vi "UHR-Fleezers Control (host) -Leonardo 04-2018 V3_greenctrl.vi"(0 "Tab Green FB":T5(tab)=enum."Trap Control (RF)") -> ()   [LabVIEW 2013] (continued)
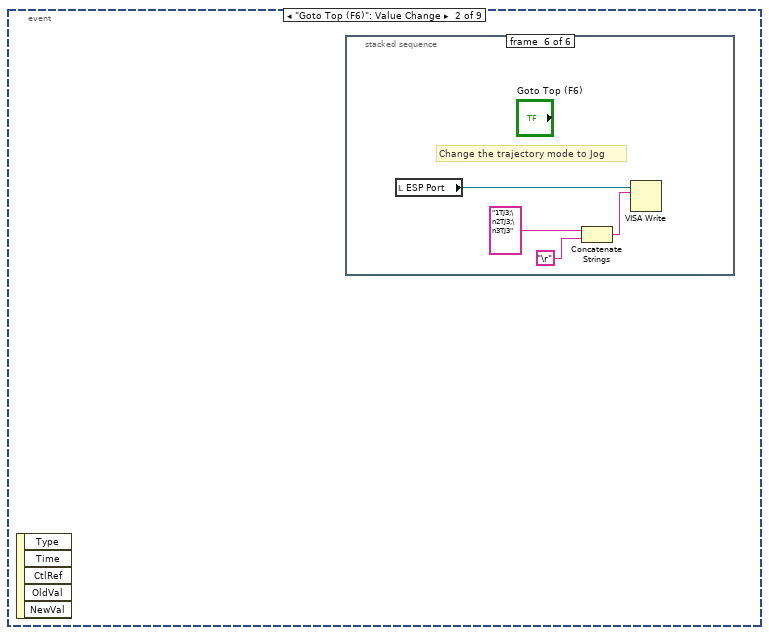
[diagram p4: hidden frame]
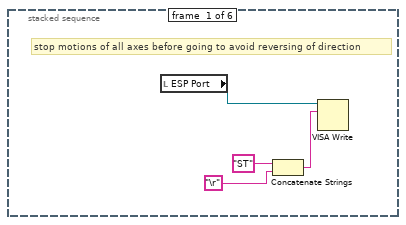
[diagram p5: hidden frame]
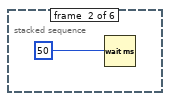
[diagram p6: hidden frame]
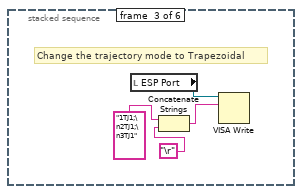
[diagram p7: hidden frame]
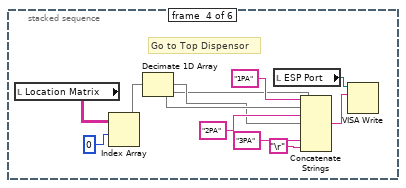
[diagram p8: hidden frame]
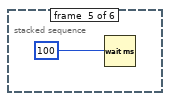
[diagram p9: hidden frame]
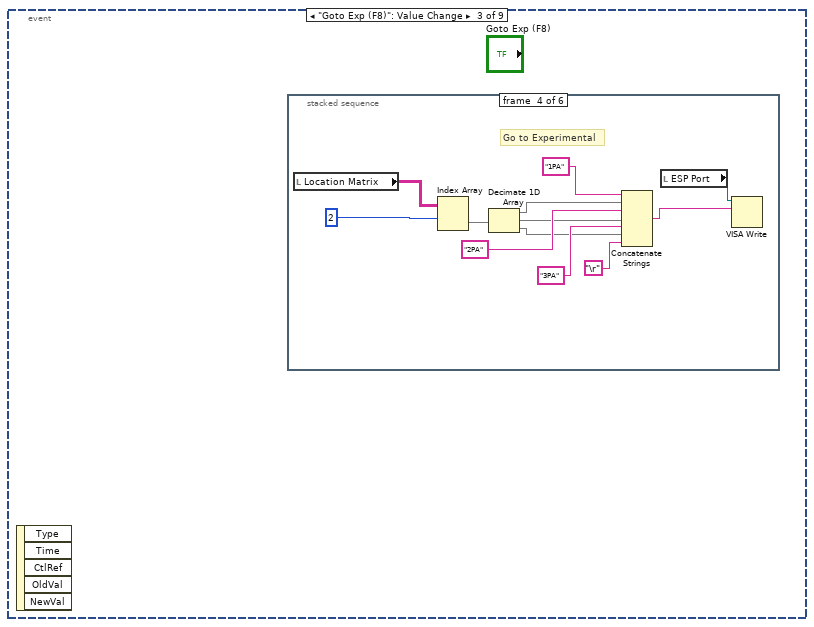
[diagram p10: hidden frame]
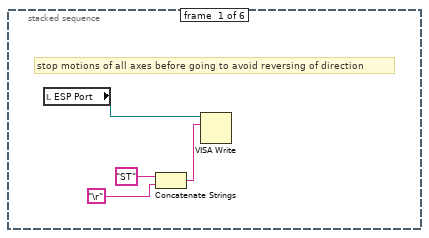
[diagram p11: hidden frame]
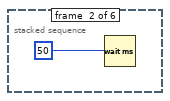
[diagram p12: hidden frame]
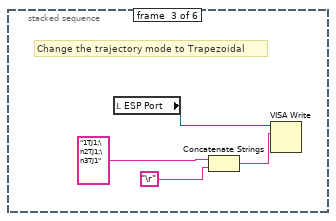
[diagram p13: hidden frame]
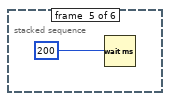
[diagram p14: hidden frame]
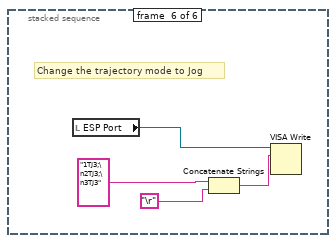
[diagram p15: hidden frame]
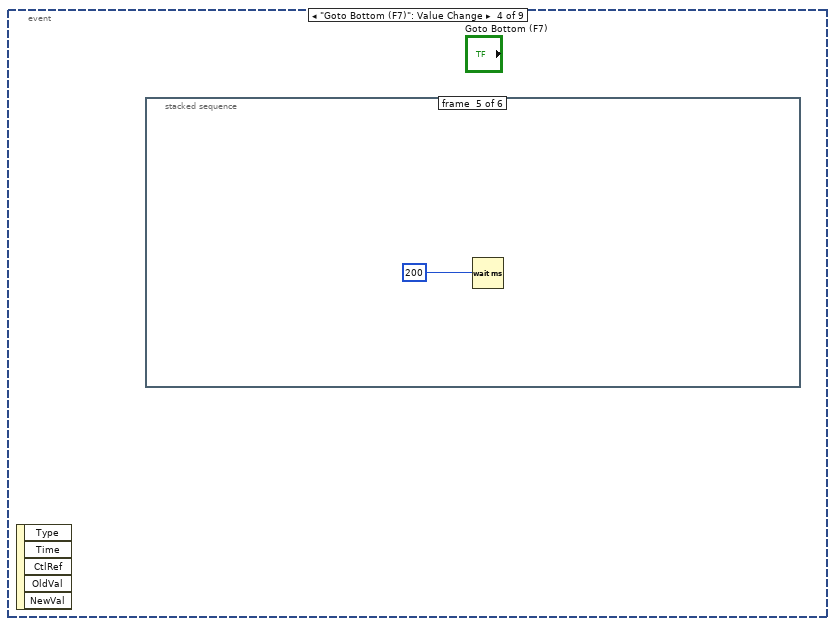
[diagram p16: hidden frame]
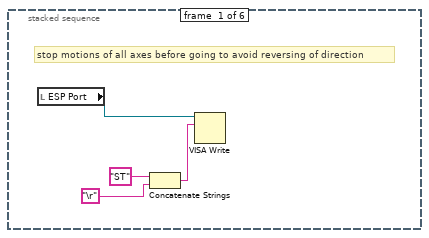
[diagram p17: hidden frame]
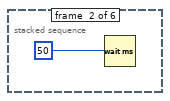
[diagram p18: hidden frame]
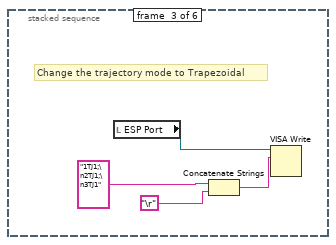
[diagram p19: hidden frame]
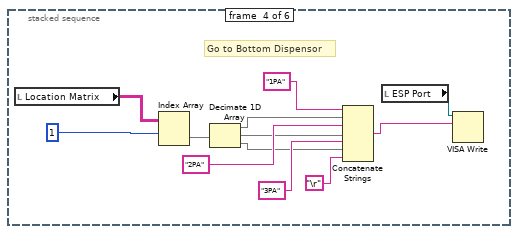
[diagram p20: hidden frame]
                  tunnel: w3888 -> [w3958 w3969]
                  tunnel: [w3958 w3961] -> w3887
                  tunnel: "Save ave N" -> [_ w3962]
                  frame False {
                  }
                  frame True {
                    w3959 = 2 ("dimension size")
                    n2326 = Array Size(array=w3969) -> (size(s)=w3963:i32)
                    n2327 = Divide(x=w3963, y=w3959) -> (x/y=w3967:dbl)
                    n2328 = Reshape Array(w3969, w3967, w3959) -> (w3968:u64[][])
                    n2329 = Transpose 2D Array(2D array=w3968) -> (transposed array=w3966:u64[][])
                    n2330 = for {
                      tunnel: w3966 -> [w3971] mode=indexing
                      tunnel: [w3970] -> w3960 mode=indexing
                      tunnel: w3962 -> [w3972]
                      workers-P: _ -> [_]
                      n2331 = call "downsample 1D array - U64.vi"("Ave N"=w3972, "Array In"=w3971) -> ("Array Out"=w3970:u64[])  [unwired: 1 in]
                    }
                    n2332 = Transpose 2D Array(2D array=w3960) -> (transposed array=w3965:u64[][])
                    n2333 = Divide(x=w3963, y=w3962) -> (x/y=w3964:dbl)
                    n2334 = Reshape Array(w3965, w3964) -> (w3961:u64[])
                  }
                }
                n2335 = case shown="True" w3889 {
                  tunnel: w3949 -> [w3981 w3993]
                  tunnel: [w3981 w3985] -> w3945
                  tunnel: "Save ave N" -> [_ w3986]
                  tunnel: w3940 -> [_ w3984]
                  frame False {
                    # "don't downsample data for trap calibration"
                  }
                  frame True {
                    n2336 = Array Size(array=w3993) -> (size(s)=w3987:i32)
                    n2337 = Array Size(array=w3984) -> (size(s)=w3983:i32)
                    n2338 = Divide(x=w3987, y=w3983) -> (x/y=w3991:dbl)
                    n2339 = Reshape Array(w3993, w3991, w3983) -> (w3992:i16[][])
                    n2340 = Transpose 2D Array(2D array=w3992) -> (transposed array=w3990:i16[][])
                    n2341 = for {
                      tunnel: w3990 -> [w3996] mode=indexing
                      tunnel: [w3995] -> w3982 mode=indexing
                      tunnel: w3986 -> [w3994]
                      workers-P: _ -> [_]
                      n2342 = call "downsample 1D array - I16.vi"("Ave N"=w3994, "Array In"=w3996) -> ("Array Out"=w3995:i16[])  [unwired: 1 out]
                    }
                    n2343 = Transpose 2D Array(2D array=w3982) -> (transposed array=w3989:i16[][])
                    n2344 = Divide(x=w3987, y=w3986) -> (x/y=w3988:dbl)
                    n2345 = Reshape Array(w3989, w3988) -> (w3985:i16[])
                  }
                }
                n2346 = Index Array(array=w3911, index=1) -> (element=w3914:waveform(dbl))
                n2347 = Index Array(array=w3911, index=0) -> (element=w3916:waveform(dbl))
                n2348 = Unbundle By Name(w3914) -> ("Y"=w3918:dbl[])
                n2349 = Unbundle By Name(w3916) -> ("Y"=w3926:dbl[])
                n2350 = case "Write trap pos. data" shown="True" w3892 {
                  tunnel: w3891 -> [_ w3974]
                  tunnel: w3887 -> [_ w3973]
                  frame False {
                  }
                  frame True {
                    n2351 = Write to Binary File(file (use dialog)=w3974, data=w3973, 5:FALSE ("prepend array or string size? (T)"), 9:T30."big-endian, network order" ("byte order (0:big-endian, network order)")) -> ()  [unwired: 1 in, 4 out]
                  }
                }
                n2352 = Write to Binary File(file (use dialog)=w3952, data=w3945, 5:FALSE ("prepend array or string size? (T)"), 9:T30."big-endian, network order" ("byte order (0:big-endian, network order)")) -> ()  [unwired: 1 in, 4 out]
                n2353 = feedback #26(w3918) -> (w3920:dbl[])
                n2354 = Build Array (concatenate)(w3920, w3918) -> (w3919:dbl[])
                n2355 = Select(t=w3918, s=w3894, f=w3919) -> (s? t:f=w3904:dbl[])
                n2356 = feedback-in #26(w3904) -> ()
                n2357 = feedback #27(w3926) -> (w3939:dbl[])
                n2358 = Build Array (concatenate)(w3939, w3926) -> (w3938:dbl[])
                n2359 = Select(t=w3926, s=w3894, f=w3938) -> (s? t:f=w3913:dbl[])
                n2360 = feedback-in #27(w3913) -> ()
                n2361 = Divide(x=w3953, y=w3954) -> (x/y=w3956:dbl)
                n2362 = Multiply(x=w3956, y=100.0) -> (x*y=w3955:dbl)
                n2363 = Build Array(w3913, w3904) -> (→"Saved APD":dbl[][])
                n2364 = Array Size(array=w3913) -> (size(s)=w3931:i32)
                n2365 = Unbundle By Name(w3933) -> ("Y"=w3937:dbl[])
                n2366 = Subtract(x=w3931, y="N pts to average") -> (x-y=w3907:i32)
                n2367 = Multiply(x="N pts to average", y=u16 2) -> (x*y=w3908:u16)
                n2368 = Subtract(x=w3931, y=w3908) -> (x-y=w3906:i32)
                n2369 = feedback #28(w3937) -> (w3936:dbl[])
                n2370 = Build Array (concatenate)(w3936, w3937) -> (w3935:dbl[])
                n2371 = Select(t=w3937, s=w3894, f=w3935) -> (s? t:f=w3934:dbl[])
                "Trap Delta Graph" <- w3934
                n2372 = feedback-in #28(w3934) -> ()
                n2373 = Array Subset(array=w3913, index=w3907, length="N pts to average") -> (w3930:dbl[])
                n2374 = Array Subset(array=w3913, index=w3906, length="N pts to average") -> (w3929:dbl[])
                n2375 = Array Subset(array=w3904, index=w3907, length="N pts to average") -> (w3910:dbl[])
                n2376 = Array Subset(array=w3904, index=w3906, length="N pts to average") -> (w3909:dbl[])
                n2377 = call-poly <vilib>:"Mean.vi"("X"=w3930) -> ("mean"=w3928:dbl)  [unwired: 1 out]
                n2378 = call-poly <vilib>:"Mean.vi"("X"=w3910) -> ("mean"=w3903:dbl)  [unwired: 1 out]
                n2379 = call-poly <vilib>:"Mean.vi"("X"=w3929) -> ("mean"=w3927:dbl)  [unwired: 1 out]
                n2380 = call-poly <vilib>:"Mean.vi"("X"=w3909) -> ("mean"=w3902:dbl)  [unwired: 1 out]
                n2381 = Subtract(x=w3903, y=w3902) -> (x-y=w3893:dbl)
                "Delta Fl. 2" <- w3893
                n2382 = Subtract(x=w3928, y=w3927) -> (x-y=w3925:dbl)
                "Delta Fl. 1" <- w3925
                n2383 = Initialize Array(w3925, 1 ("dimension size")) -> (w3922:dbl[])
                n2384 = Initialize Array(w3893, 1 ("dimension size")) -> (w3899:dbl[])
                n2385 = feedback #29(w3922) -> (w3923:dbl[])
                n2386 = Build Array (concatenate)(w3923, w3922) -> (w3921:dbl[])
                n2387 = feedback #30(w3899) -> (w3900:dbl[])
                n2388 = Build Array (concatenate)(w3900, w3899) -> (w3898:dbl[])
                n2389 = Select(t=w3922, s=w3894, f=w3921) -> (s? t:f=w3897:dbl[])
                n2390 = feedback-in #29(w3897) -> ()
                n2391 = Select(t=w3899, s=w3894, f=w3898) -> (s? t:f=w3896:dbl[])
                n2392 = feedback-in #30(w3896) -> ()
                n2393 = Build Array(w3897, w3896) -> (→"Save APD Deriv":dbl[][])
              }
            }
            "Progress" <- w3870
            "Progress 2" <- w3870
          }
        }
      }
    }
    n2394 = Divide(x=w2251, y=w2252) -> (x/y=w2242:ext)
    "Trap 2 amplitude" <- w2242
    n2395 = Bundle By Name(cluster=w2505, "Green FB Ch 0"=w2504, "Green FB Ch 1"=w2503) -> (w2489:T49)
    "Green FB Signals (V)" <- w2489
    n2396 = case shown="True" w2244 {
      tunnel: w2243 -> [_ w2594]
      tunnel: w2242 -> [_ w2593]
      frame False {
      }
      frame True {
        w2595 = 50.0
        n2397 = Greater?(x=w2593, y=w2595) -> (0:w2591:bool)
        n2398 = Greater?(x=w2594, y=w2595) -> (0:w2592:bool)
        n2399 = Or(x=w2592, y=w2591) -> (x .or. y?=w2590:bool)
        n2400 = case shown="True" w2590 {
          frame False {
          }
          frame True {
            n2401 = property on="All FB On/Off" class="Bool (strict)"("Val(Sgnl)"=FALSE) -> ()  [unwired: 2 in, 2 out]
            "Feedback overload" <- TRUE
          }
        }
      }
    }
    n2402 = Unbundle By Name(w2489) -> ("Green FB Ch 2"=→"Green FB Plot":dbl)
    n2403 = local read "wait to reset values"() -> (w2573:bool)
    n2404 = Not(x=w2570) -> (.not. x?=w2574:bool)
    n2405 = And(x=w2574, y=w2573) -> (x .and. y?=w2575:bool)
    n2406 = case "Part of MCL raster scanning: returns to initial positions after scan done" shown="True" w2575 {
      tunnel: w2578 -> [w3419 w3426]
      tunnel: [w3419 w3425] -> w2577
      tunnel: w2572 -> [w3418 w3424]
      tunnel: [w3418 w3423] -> w2571
      frame False {
      }
      frame True {
        w3434 = 10.0 ("y")
        w3433 = 32767.0 ("y")
        # "to return scan values\nafter a synchronous \nAOM scan"
        n2407 = local read "AO2"() -> (w3427:dbl)
        n2408 = local read "AO1"() -> (w3428:dbl)
        n2409 = local write "wait to reset values"(FALSE ("wait to reset values")) -> ()
        n2410 = Multiply(x=w3428, y=w3433) -> (x*y=w3430:dbl)
        n2411 = Multiply(x=w3427, y=w3433) -> (x*y=w3432:dbl)
        n2412 = Divide(x=w3430, y=w3434) -> (x/y=w3429:dbl)
        n2413 = Divide(x=w3432, y=w3434) -> (x/y=w3431:dbl)
        n2414 = To Word Integer(number=w3429) -> (16bit integer=w3435:i16)
        n2415 = To Word Integer(number=w3431) -> (16bit integer=w3436:i16)
        n2416 = local read "Total Counts (ticks)"() -> (w3420:u32)
        n2417 = xnode "Read/Write Control"("FPGA VI Reference In"=w3426, "error in"=w3424, "AO1 (Y)"=w3435, "AO2 (X)"=w3436, "MCL count"=w3420) -> ("FPGA VI Reference Out"=w3425:T20, "error out"=w3423:errorcluster)
        n2418 = local read "Scan Range (V)\n(of steps)"() -> (w3421:dbl)
        n2419 = property on="Scan Range (V)\n(of steps)" class="DigNum (strict)"("Val(Sgnl)"=w3421) -> ()  [unwired: 2 in, 2 out]
      }
    }
    n2420 = node-c288() -> ()  [unwired: 2 out]
  }
  n2421 = node-c288(3 ("Processor")) -> (w108:T25)  [unwired: 3 out]
  n2422 = timed-loop "Oscillate AOD (debugging)" {
    tunnel: w61 -> [w3998]
    tunnel: [w3997] -> w72
    timing: w108 -> [_]
    timing-out: [_] -> w107
    stop <- w3997 stop-if-true
    n2423 = node-c288() -> ()  [unwired: 2 out]
    n2424 = event shown="[0] \"Oscillate Set 2\", \"Fish for Tether\": Value Change" {
      selector: _ -> [_ _ _]
      dyn-events: _ -> [_ _ _]
      timeout: _ -> [_ _ _]
      tunnel: w3998 -> [w4005 _ _]
      tunnel: [FALSE ("Stop All") _ w4273] -> w3997
      event "Oscillate Set 2", "Fish for Tether": Value Change {
        n2425 = event-data() -> ()  [unwired: 6 out]
        n2426 = local read "Oscillate Set 2"() -> (w4004:bool)
        n2427 = Or(x=w4004, y="Fish for Tether") -> (x .or. y?=w4002:bool)
        n2428 = case shown="True" w4002 {
          tunnel: w4005 -> [_ w4008]
          tunnel: "Fish for Tether" -> [_ w4007]
          frame False {
          }
          frame True {
            n2429 = case shown="True" w4007 {
              frame False {
              }
              frame True {
                n2430 = local write "Scan axis 2"(TRUE) -> ()
                n2431 = local write "Tether"(FALSE ("Tether")) -> ()
              }
            }
            n2432 = node-c288("Period") -> (w4010:T25)  [unwired: 3 out]
            n2433 = timed-loop "Oscillate AOD" {
              timing: w4010 -> [_]
              timing-out: [_] -> w4009
              tunnel: w4008 -> [w4020]
              tunnel: w4007 -> [w4019]
              i -> [w4022]
              stop <- w4018 stop-if-true
              n2434 = node-c288() -> (w4021:i64)  [unwired: 1 out]
              n2435 = flat-sequence {
                tunnel: w4022 -> [w4048]
                tunnel: w4021 -> [w4047]
                tunnel: w4020 -> [w4031]
                tunnel: w4019 -> [w4033]
                tunnel: [w4033] -> w4017
                tunnel: [w4032] -> w4016
                tunnel: [w4030] -> w4015
                tunnel: [w4027] -> w4013
                tunnel: w4017 -> [w4084]
                tunnel: w4016 -> [w4082]
                tunnel: w4015 -> [w4081]
                tunnel: [w4080] -> w4014
                tunnel: w4013 -> [w4079]
                tunnel: [w4148] -> w4018
                tunnel: w4014 -> [w4146]
                frame #0 {
                  n2436 = Divide(x=w4047, y=i64 1000) -> (x/y=w4042:dbl)
                  n2437 = Multiply(x=w4042, y=w4048) -> (x*y=w4044:dbl)
                  n2438 = Multiply(x="Osc. freq. (Hz)", y=6.283185307179586) -> (x*y=w4045:dbl)
                  n2439 = Multiply(x=w4045, y=w4044) -> (x*y=w4029:dbl)
                  n2440 = local read "BD 1 Frequency 2 (MHz)"() -> (w4026:dbl)
                  n2441 = local read "BD 1 Frequency 1 (MHz)"() -> (w4023:dbl)
                  n2442 = case shown="True" w4033 {
                    tunnel: w4029 -> [w4054 w4061]
                    tunnel: w4026 -> [_ w4071]
                    tunnel: [w4051 w4055] -> w4034
                    tunnel: [FALSE w4064] -> w4030
                    tunnel: [0.0 w4057] -> w4027
                    tunnel: w4023 -> [_ w4056]
                    frame False {
                      n2443 = Sine(x=w4054) -> (sin(x)=w4052:dbl)
                      n2444 = Multiply(x=w4052, y="Osc. amp. (MHz)") -> (x*y=w4051:dbl)
                    }
                    frame True {
                      n2445 = Cosine(x=w4061) -> (cos(x)=w4074:dbl)
                      n2446 = Subtract(x=w4071, y=w4056) -> (x-y=w4070:dbl)
                      n2447 = Decrement(x=w4074) -> (x-1=w4073:dbl)
                      n2448 = Subtract(x=w4070, y="Closest Delta (MHz)") -> (x-y=w4067:dbl)
                      n2449 = Divide(x=w4073, y=2.0) -> (x/y=w4068:dbl)
                      n2450 = Multiply(x=w4068, y=w4067) -> (x*y=w4055:dbl)
                      n2451 = local read "Vec Mean of T1 T2"() -> (w4063:dbl[])
                      n2452 = Greater?(x=w4063, y="Stop F (pN)") -> (0:w4065:bool[])
                      n2453 = Or Array Elements(Boolean array=w4065) -> (logical OR=w4064:bool)
                      n2454 = Divide(x=w4061, y=6.283185307179586) -> (x/y=w4060:dbl)
                      n2455 = Round Toward +Infinity(x=w4060) -> (ceil(x): smallest int >= x=w4057:dbl)
                      "Attempts" <- w4057
                      n2456 = Greater?(x=w4057, y="Attempt Limit") -> (0:w4059:bool)
                      n2457 = case shown="True" w4059 {
                        frame False {
                        }
                        frame True {
                          n2458 = local write "Fish for Tether"(FALSE ("Fish for Tether")) -> ()
                          n2459 = call <vilib>:"Beep.vi"() -> ()  [unwired: 3 in, 9 out]
                          n2460 = local read "Messages"() -> (w4076:string)
                          n2461 = call "Update messages.vi"("Message to add"="Tether fishing timeout." ("Messages"), "Old message string"=w4076) -> ("New message string"=→"Messages":string)
                        }
                      }
                    }
                  }
                  n2462 = local read "Y RF Frequency Limits (MHz)"() -> (w4035:T16)
                  n2463 = local read "X RF Frequency Limits (MHz)"() -> (w4036:T16)
                  n2464 = local read "BD 1 Frequency 3 (MHz)"() -> (w4041:dbl)
                  n2465 = local read "BD 2 Frequency 2 (MHz)"() -> (w4025:dbl)
                  n2466 = Select(t=w4026, s="Scan axis 2", f=w4025) -> (s? t:f=w4037:dbl)
                  n2467 = Add(x=w4034, y=w4037) -> (x+y=w4032:dbl)
                  n2468 = Select(t=w4032, s="Scan axis 2", f=w4026) -> (s? t:f=w4024:dbl)
                  n2469 = Select(t=w4025, s="Scan axis 2", f=w4032) -> (s? t:f=w4039:dbl)
                  n2470 = local read "BD 2 Frequency 3 (MHz)"() -> (w4040:dbl)
                  n2471 = call "set RF board frequency - interlace.vi"("Board 2 Frequency Limits"=w4035, "Board 1 Frequency Limits"=w4036, "FPGA VI Reference In"=w4031, "Board 2 Frequency 3 (MHz)"=w4040, "Board 1 Frequency 3 (MHz)"=w4041, "Board 2 Frequency 2 (MHz)"=w4025, "Board 2 Frequency 1 (MHz)"=w4039, "Board 1 Frequency 2 (MHz)"=w4024, "Board 1 Frequency 1  (MHz)"=w4023) -> ()  [unwired: 1 in, 2 out]
                }
                frame #1 {
                  n2472 = And(x=w4084, y=w4081) -> (x .and. y?=w4083:bool)
                  n2473 = case "Only if were fishing and now formed tether" shown="True" w4083 {
                    tunnel: w4082 -> [w4086 w4098]
                    tunnel: [w4085 w4097] -> w4080
                    tunnel: w4079 -> [_ w4093]
                    frame False {
                      n2474 = local read "Fish for Tether"() -> (w4085:bool)
                      n2475 = case shown="True" w4085 {
                        tunnel: w4086 -> [_ _]
                        frame False {
                        }
                        frame True {
                        }
                      }
                    }
                    frame True {
                      w4097 = FALSE ("Fish for Tether")
                      n2476 = call <vilib>:"Beep.vi"() -> ()  [unwired: 3 in, 9 out]
                      n2477 = Number To Decimal String(number=w4093, width (-)=i16 1) -> (decimal integer string=w4091:string)
                      n2478 = case shown="\"2\", \"3\", \"4\", \"5\", \"6\"" "Then..." {
                        selector: "Then..." -> [_ w4101]
                        tunnel: w4098 -> [w4100 _]
                        frame "1", Default {
                          # "do nothing"
                          n2479 = property on="BD 1 Frequency 1 (MHz)" class="DigNum (strict)"("Val(Sgnl)"=w4100) -> ()  [unwired: 2 in, 2 out]
                        }
                        frame "2", "3", "4", "5", "6" {
                          n2480 = flat-sequence {
                            tunnel: w4101 -> [w4103]
                            frame #0 {
                              n2481 = property on="Trap Delta (MHz)" class="DigNum (strict)"("Val(Sgnl)"="Move to Delta 1 (MHz)") -> ()  [unwired: 2 in, 2 out]
                            }
                            frame #1 {
                              n2482 = case shown="\"5\", \"6\"" w4103 {
                                selector: w4103 -> [w4106 w4116 _]
                                frame "3", "4" {
                                n2483 = flat-sequence {
                                tunnel: w4106 -> [w4107]
                                tunnel: [w4107] -> w4104
                                tunnel: [w4109] -> w4105
                                tunnel: w4104 -> [w4109]
                                tunnel: w4105 -> [w4113]
                                frame #0 {
                                n2484 = property on="Green Laser ON/Interlacing" class="Bool (strict)"("Val(Sgnl)"=TRUE ("Value (Signaling)")) -> ()  [unwired: 2 in, 2 out]
                                }
                                frame #1 {
                                n2485 = Multiply(x="Wait Before Save (s)", y=u32 1000 ("x")) -> (x*y=w4111:u32)
                                n2486 = Wait (ms)(milliseconds to wait=w4111) -> ()  [unwired: 1 out]
                                }
                                frame #2 {
                                n2487 = property on="Start Saving" class="Bool (strict)"("Value"=TRUE ("Start Saving")) -> ()  [unwired: 2 in, 2 out]
                                n2488 = case shown="Default" w4113 {
                                frame Default {
                                }
                                frame "4" {
                                n2489 = property on="Fl. Triggered..." class="Bool (strict)"("Val(Sgnl)"=TRUE ("Value (Signaling)")) -> ()  [unwired: 2 in, 2 out]
                                }
                                }
                                }
                                }
                                }
                                frame "5", "6" {
                                n2490 = stacked-sequence {
                                tunnel: w4116 -> [_ _ _ _ _ _ _ _ w4133 _ _]
                                frame #0 {
                                n2491 = Replace Array Subset(array=u32[] [0] ("Index Values"), new element="Raster Set Upon Tether", index=0) -> (w4117:u32[])
                                n2492 = property on="Saved AOD Raster Scan Parameter Sets" class="Arr (strict)"("Index Values"=w4117) -> ()  [unwired: 2 in, 2 out]
                                }
                                frame #1 {
                                n2493 = Wait (ms)(milliseconds to wait=u32 500) -> ()  [unwired: 1 out]
                                }
                                frame #2 {
                                n2494 = property on="Load parameters" class="Bool (strict)"("Val(Sgnl)"=TRUE ("Value (Signaling)")) -> ()  [unwired: 2 in, 2 out]
                                }
                                frame #3 {
                                n2495 = Wait (ms)(milliseconds to wait=u32 500) -> ()  [unwired: 1 out]
                                }
                                frame #4 {
                                n2496 = property on="Trap Raster Scan" class="Bool (strict)"("Val(Sgnl)"=TRUE ("Value (Signaling)")) -> ()  [unwired: 2 in, 2 out]
                                }
                                frame #5 {
                                n2497 = Wait (ms)(milliseconds to wait=u32 2000) -> ()  [unwired: 1 out]
                                }
                                frame #6 {
                                n2498 = while {
                                stop <- w4128 stop-if-true
                                n2499 = local read "Raster Scanning..."() -> (w4127:bool)
                                n2500 = local read "Saving..."() -> (w4130:bool)
                                n2501 = Wait (ms)(milliseconds to wait=u32 100) -> ()  [unwired: 1 out]
                                n2502 = Not(x=w4130) -> (.not. x?=w4129:bool)
                                n2503 = Not(x=w4127) -> (.not. x?=w4126:bool)
                                n2504 = And(x=w4129, y=w4126) -> (x .and. y?=w4128:bool)
                                }
                                }
                                frame #7 {
                                n2505 = property on="Trap Delta (MHz)" class="DigNum (strict)"("Val(Sgnl)"="Move to Delta 2 (MHz)") -> ()  [unwired: 2 in, 2 out]
                                }
                                frame #8 {
                                n2506 = local read "Tether"() -> (w4134:bool)
                                n2507 = case shown="True" w4134 {
                                tunnel: w4133 -> [_ w4135]
                                frame False {
                                }
                                frame True {
                                n2508 = flat-sequence {
                                tunnel: w4135 -> [w4137]
                                frame #0 {
                                n2509 = Wait (ms)(milliseconds to wait=u32 500) -> ()  [unwired: 1 out]
                                }
                                frame #1 {
                                n2510 = case shown="\"6\"" w4137 {
                                frame Default {
                                }
                                frame "6" {
                                n2511 = property on="Green Laser ON/Interlacing" class="Bool (strict)"("Val(Sgnl)"=TRUE ("Green Laser ON/Interlacing")) -> ()  [unwired: 2 in, 2 out]
                                }
                                }
                                }
                                frame #2 {
                                n2512 = Wait (ms)(milliseconds to wait=u32 500) -> ()  [unwired: 1 out]
                                }
                                frame #3 {
                                n2513 = local write "Start Saving"("Save at end (5, 6)") -> ()
                                }
                                }
                                }
                                }
                                }
                                frame #9 {
                                n2514 = local read "Bead Sep. Int. Time (s)"() -> (w4143:dbl)
                                n2515 = Multiply(x=w4143, y=1000.0) -> (x*y=w4142:dbl)
                                n2516 = Wait (ms)(milliseconds to wait=w4142) -> ()  [unwired: 1 out]
                                }
                                frame #10 {
                                n2517 = property on="Rescale on Mean" class="Bool (strict)"("Val(Sgnl)"=TRUE ("Value (Signaling)")) -> ()  [unwired: 2 in, 2 out]
                                }
                                }
                                }
                                frame "2", Default {
                                }
                              }
                            }
                          }
                        }
                      }
                      n2518 = Concatenate Strings("Formed tether in ", w4091, " attempt(s)." ("string")) -> (w4088:string)
                      n2519 = local read "Messages"() -> (w4095:string)
                      n2520 = local write "Fish for Tether"(w4097) -> ()
                      n2521 = call "Update messages.vi"("Message to add"=w4088, "Old message string"=w4095) -> ("New message string"=w4094:string)
                      n2522 = local write "Messages"(w4094) -> ()
                      n2523 = Get Date/Time In Seconds() -> (seconds since 1Jan1904=→"Time tether formed":timestamp)
                      "Tether" <- "Tether Alarm?"
                    }
                  }
                }
                frame #2 {
                  n2524 = local read "Oscillate Set 2"() -> (w4147:bool)
                  n2525 = local read "Stop All"() -> (w4149:bool)
                  n2526 = Not Or(1:w4146, 2:w4147) -> (0:w4145:bool)
                  n2527 = Compound Arithmetic op=OR(w4149, w4145) -> (w4148:bool)
                }
              }
              n2528 = node-c288() -> ()  [unwired: 2 out]
            }
            n2529 = node-c288(w4009) -> ()  [unwired: 1 out]
          }
        }
      }
      event "Fl. Triggered...": Value Change {
        n2530 = event-data() -> ()  [unwired: 7 out]
        n2531 = case shown="True" "Fl. Triggered..." {
          frame False {
          }
          frame True {
            n2532 = node-c288() -> (w4161:T25)  [unwired: 4 out]
            n2533 = timed-loop {
              timing: w4161 -> [_]
              timing-out: [_] -> w4160
              tunnel: "Action" -> [w4165]
              shift-right: [w4162] -> _
              shift-left: u8 255 -> [w4164]
              stop <- w4166 stop-if-true
              n2534 = node-c288() -> ()  [unwired: 2 out]
              n2535 = flat-sequence {
                tunnel: w4165 -> [w4178]
                tunnel: w4164 -> [w4175]
                tunnel: [w4174] -> w4163
                tunnel: [w4264] -> w4166
                tunnel: w4163 -> [w4263]
                tunnel: [w4263] -> w4162
                frame #0 {
                  n2536 = local read "Delta Fl. 2"() -> (w4169:dbl)
                  n2537 = local read "Delta Fl. 1"() -> (w4170:dbl)
                  n2538 = Select(t=w4170, s="APD to Watch", f=w4169) -> (s? t:f=w4168:dbl)
                  n2539 = Multiply(x="Fl. Delta Thresh. (kHz)", y=1000.0) -> (x*y=w4177:dbl)
                  n2540 = Greater?(x=w4168, y=w4177) -> (0:w4172:bool)
                  n2541 = Or(x="Force Yank", y=w4172) -> (x .or. y?=w4173:bool)
                  n2542 = case shown="True" w4173 {
                    tunnel: w4178 -> [_ w4188]
                    tunnel: w4175 -> [w4180 w4184]
                    tunnel: [w4180 w4181] -> w4174
                    frame False {
                    }
                    frame True {
                      n2543 = flat-sequence {
                        tunnel: w4185 -> [w4194]
                        tunnel: [w4194] -> w4189
                        tunnel: w4188 -> [w4193]
                        tunnel: [w4193] -> w4187
                        tunnel: [w4192] -> w4186
                        tunnel: w4184 -> [w4191]
                        tunnel: [w4190] -> w4183
                        tunnel: w4189 -> [w4219]
                        tunnel: w4187 -> [w4218]
                        tunnel: w4186 -> [w4217]
                        tunnel: w4183 -> [w4216]
                        tunnel: [w4216] -> w4182
                        tunnel: w4182 -> [w4261]
                        tunnel: [w4261] -> w4181
                        frame #0 {
                          n2544 = call <vilib>:"Beep.vi"() -> ()  [unwired: 3 in, 9 out]
                          n2545 = local write "Waiting"(FALSE ("Waiting")) -> ()
                          n2546 = Increment(x=w4191) -> (x+1=w4190:u8)
                          n2547 = case shown="\"Yank\"" w4193 {
                            tunnel: w4190 -> [_ _ w4200]
                            frame "Image" {
                              n2548 = property on="Confocal Image" class="Bool (strict)"("Val(Sgnl)"=TRUE ("Value (Signaling)")) -> ()  [unwired: 2 in, 2 out]
                            }
                            frame "Alarm", Default {
                            }
                            frame "Yank" {
                              n2549 = flat-sequence {
                                tunnel: w4200 -> [w4203]
                                tunnel: [w4202] -> w4199
                                tunnel: ["N Array El"] -> w4198
                                tunnel: w4199 -> [w4213]
                                tunnel: w4198 -> [w4209]
                                frame #0 {
                                n2550 = Multiply(x="Yank Delay (s)", y=1000.0) -> (x*y=w4206:dbl)
                                n2551 = Quotient & Remainder(x=w4203, y="N Array El") -> (x-y*floor(x/y)=w4202:u8)  [unwired: 1 out]
                                n2552 = Wait (ms)(milliseconds to wait=w4206) -> ()  [unwired: 1 out]
                                }
                                frame #1 {
                                n2553 = Random Number (0-1)() -> (number: 0 to 1=w4210:dbl)
                                n2554 = Multiply(x=w4209, y=w4210) -> (x*y=w4208:dbl)
                                n2555 = Round Toward -Infinity(1:w4208) -> (0:w4207:dbl)
                                n2556 = Select(t=w4207, s="Random Choice", f=w4213) -> (s? t:f=w4211:dbl)
                                n2557 = Index Array(array="Yank to Delta Array (MHz)", index=w4211) -> (element=w4214:dbl)
                                n2558 = property on="Trap Delta (MHz)" class="DigNum (strict)"("Val(Sgnl)"=w4214) -> ()  [unwired: 2 in, 2 out]
                                }
                              }
                            }
                          }
                          n2559 = local read "Time (s)"() -> (w4192:dbl)
                          "Fl. High" <- TRUE ("Yanking")
                        }
                        frame #1 {
                          n2560 = node-c288() -> (w4221:T25)  [unwired: 4 out]
                          n2561 = timed-loop {
                            timing: w4221 -> [_]
                            timing-out: [_] -> w4220
                            tunnel: w4219 -> [w4237]
                            tunnel: w4218 -> [w4235]
                            tunnel: w4217 -> [w4234]
                            stop <- w4236 stop-if-true
                            n2562 = node-c288() -> ()  [unwired: 2 out]
                            n2563 = local read "Fl. Delta Thresh. (kHz)"() -> (w4229:dbl)
                            n2564 = local read "Fl. Triggered..."() -> (w4238:bool)
                            n2565 = local read "Delta Fl. 1"() -> (w4225:dbl)
                            n2566 = local read "Delta Fl. 2"() -> (w4223:dbl)
                            n2567 = local read "Stop All"() -> (w4232:bool)
                            n2568 = local read "APD to Watch"() -> (w4224:bool)
                            n2569 = Select(t=w4225, s=w4224, f=w4223) -> (s? t:f=w4222:dbl)
                            n2570 = Not(x=w4238) -> (.not. x?=w4233:bool)
                            n2571 = Multiply(x=w4229, y=1000.0) -> (x*y=w4228:dbl)
                            n2572 = Negate(x=w4228) -> (-x=w4227:dbl)
                            n2573 = Less?(x=w4222, y=w4227) -> (x < y?=w4231:bool)
                            n2574 = Compound Arithmetic op=OR(w4231, w4232, w4233, "Force Reset") -> (w4236:bool)
                            n2575 = case shown="True" w4236 {
                              tunnel: w4237 -> [_ w4249]
                              tunnel: w4235 -> [_ w4248]
                              tunnel: w4234 -> [_ w4246]
                              frame False {
                              }
                              frame True {
                                n2576 = case shown="\"Yank\"" w4248 {
                                tunnel: w4249 -> [_ w4250]
                                frame "Image", Default {
                                }
                                frame "Yank" {
                                n2577 = flat-sequence {
                                tunnel: [w4255] -> w4251
                                tunnel: w4250 -> [w4255]
                                tunnel: w4251 -> [w4256]
                                frame #0 {
                                n2578 = local read "Yank Delay (s)"() -> (w4254:dbl)
                                n2579 = Multiply(x=w4254, y=1000.0) -> (x*y=w4252:dbl)
                                n2580 = Wait (ms)(milliseconds to wait=w4252) -> ()  [unwired: 1 out]
                                }
                                frame #1 {
                                n2581 = property on="Trap Delta (MHz)" class="DigNum (strict)"("Val(Sgnl)"=w4256) -> ()  [unwired: 2 in, 2 out]
                                }
                                }
                                }
                                }
                                n2582 = local read "Time (s)"() -> (w4247:dbl)
                                n2583 = Subtract(x=w4247, y=w4246) -> (x-y=w4243:dbl)
                                "Duration (s)" <- w4243
                                n2584 = Number To Decimal String(number=w4243, width (-)=i16 0) -> (decimal integer string=w4241:string)
                                n2585 = Concatenate Strings(w4241, " s fluorescence event." ("string")) -> (w4239:string)
                                n2586 = local read "Messages"() -> (w4245:string)
                                n2587 = call "Update messages.vi"("Message to add"=w4239, "Old message string"=w4245) -> ("New message string"=w4244:string)
                                n2588 = call <vilib>:"Beep.vi"() -> ()  [unwired: 3 in, 9 out]
                                n2589 = local write "Messages"(w4244) -> ()
                              }
                            }
                            n2590 = node-c288() -> ()  [unwired: 2 out]
                          }
                          n2591 = node-c288(w4220) -> ()  [unwired: 1 out]
                        }
                        frame #2 {
                          n2592 = local write "Fl. High"(FALSE ("Yanking")) -> ()
                        }
                      }
                      n2593 = local read "Trap Delta (MHz)"() -> (w4185:dbl)
                    }
                  }
                }
                frame #1 {
                  n2594 = local read "Stop All"() -> (w4267:bool)
                  n2595 = local read "Fl. Triggered..."() -> (w4265:bool)
                  n2596 = Not(x=w4265) -> (.not. x?=w4266:bool)
                  n2597 = Or(x=w4266, y=w4267) -> (x .or. y?=w4264:bool)
                  n2598 = Not(x=w4264) -> (.not. x?=→"Waiting":bool)
                }
              }
              n2599 = node-c288() -> ()  [unwired: 2 out]
            }
            n2600 = node-c288(w4160) -> ()  [unwired: 1 out]
          }
        }
      }
      event "Stop All": Value Change {
        n2601 = event-data() -> ()  [unwired: 7 out]
        n2602 = local read "Stop All"() -> (w4273:bool)
      }
    }
    n2603 = node-c288() -> ()  [unwired: 2 out]
  }
  n2604 = node-c288(w107) -> ()  [unwired: 1 out]
  n2605 = node-c288(w194) -> ()  [unwired: 1 out]
  n2606 = flat-sequence "@Alex - Set stage to 0,0,0 on exit" {
    tunnel: w2 -> [w4275]
    tunnel: [w4274] -> w1
    frame #0 {
      n2607 = local read "ESP Port"() -> (w4279:refnum<visa-resource-name>)
      n2608 = Concatenate Strings("1PA0;\n2PA0;\n3PA0" ("write buffer"), "\r") -> (w4276:string)
      n2609 = VISA Write(VISA resource name=w4279, write buffer=w4276, error in (no error)=w4275) -> (error out=w4274:errorcluster)  [unwired: 2 out]
    }
  }
  n2610 = flat-sequence {
    tunnel: w69 -> [w4284]
    tunnel: [w4283] -> w75
    tunnel: [w4280] -> w74
    tunnel: w73 -> [_]
    tunnel: w72 -> [_]
    tunnel: w71 -> [_]
    tunnel: w70 -> [_]
    tunnel: w1 -> [w4281]
    tunnel: w75 -> [w4287]
    tunnel: w74 -> [w4286]
    frame #0 {
      w4282 = FALSE ("APD to FIFO")
      n2611 = xnode "Read/Write Control"("FPGA VI Reference In"=w4284, "error in"=w4281, "APD to FIFO"=w4282, "AI to FIFO"=w4282) -> ("FPGA VI Reference Out"=w4283:T20, "error out"=w4280:errorcluster)
    }
    frame #1 {
      n2612 = xnode "Invoke Method"("FPGA VI Reference In"=w4287, "error in"=w4286) -> ("FPGA VI Reference Out"=w4285:T20)  [unwired: 1 out]
      n2613 = xnode "Close FPGA VI Reference"("FPGA VI Reference In"=w4285) -> ()  [unwired: 1 in, 1 out]
    }
  }
